vi "Test Find Chessboard Corners.vi"(8 "error in (no error)":errorcluster, 11 "Test Case In":refnum<class "CameraCalibration.lvclass">) -> (0 "error out":errorcluster, 3 "Test Case Out":refnum<class "CameraCalibration.lvclass">)   [LabVIEW 2020, in "g_ar_toolkit.test.lvlib" / "CameraCalibration.lvclass"]
uses:
  CameraCalibration.lvclass
  C:/Program Files (x86)/National Instruments/LabVIEW 2020/vi.lib/Astemes/LUnit/Test Case.lvclass
  g_ar_toolkit.common/Image Point (Float).ctl
  g_ar_toolkit.common/Image Size (Integer).ctl
  g_ar_toolkit.feature_detection/Chessboard Corner Info.ctl
  g_ar_toolkit.image/Interpolation Mode.ctl
  <vilib>/Astemes/LUnit/Test Case.lvclass/Test Case.ctl
  g_ar_toolkit.common/Termination Criteria/Termination Criteria.lvclass/Termination Criteria.ctl
  g_ar_toolkit.image/New Image (Greyscale).vi
  g_ar_toolkit.image/Copy Pixmap to Image (Greyscale Flatten Mask).vi
  g_ar_toolkit.image/Resize (Greyscale).vi
  g_ar_toolkit.feature_detection/FindChessboardCornersGreyscale.vi
  g_ar_toolkit.image/Draw Circle (Greyscale).vi
  g_ar_toolkit.image/Draw Image to Picture (Greyscale).vi
  g_ar_toolkit.image/New Image (Greyscale).vi/6598b9e0-8a08-46f5-91fd-ca1b87217137.vi
  g_ar_toolkit.image/Copy Pixmap to Image (Greyscale Flatten Mask).vi/f0818824-bd55-4656-87f2-fcc208e7cf24.vi
  g_ar_toolkit.image/Resize (Greyscale).vi/eaa3f26c-b51e-4a69-9610-cf2aa5919b39.vi
  g_ar_toolkit.feature_detection/FindChessboardCornersGreyscale.vi/ca99938f-1423-42fb-b653-ffd1f73e2bb5.vi
  <vilib>/Astemes/LUnit/Append Fail Result.vi
  <vilib>/Astemes/LUnit/Append Pass Result.vi
  g_ar_toolkit.common/Termination Criteria/Get Values.vi
  g_ar_toolkit.image/Draw Circle (Greyscale).vi/8336a1cf-e433-4bea-8080-376bdb783d4e.vi
  g_ar_toolkit.image/Draw Image to Picture (Greyscale).vi/9ae995ca-ccda-485c-89ac-02736fde3e8e.vi
  g_ar_toolkit.image/FixPixmap.vi
  <vilib>/Astemes/LUnit/Run In UI.vi
  g_ar_toolkit.image/Default8bitColourMap.vi
  <vilib>/Utility/error.llb/Clear Errors.vi
  <vilib>/picture/picture.llb/Draw Rectangle.vi
  <vilib>/picture/pictutil.llb/Picture to Pixmap.vi
  g_ar_toolkit.common/Module Path.vi
  <vilib>/Utility/error.llb/Error Cluster From Error Code.vi
  g_ar_toolkit.common/Termination Criteria/Termination Criteria.lvclass
  CameraCalibration.lvclass/CameraCalibration.ctl
  g_ar_toolkit.image/g_ar_toolkit.image.lvlib
  g_ar_toolkit.feature_detection/g_ar_toolkit.feature_detection.lvlib
  <vilib>/Astemes/LUnit/Test Case.lvclass
  g_ar_toolkit.common/g_ar_toolkit.common.lvlib
panel:
  out "Points":T1[](array[typedef])
  out "Points Refined":T1[](array[typedef])
  out "Picture":picture
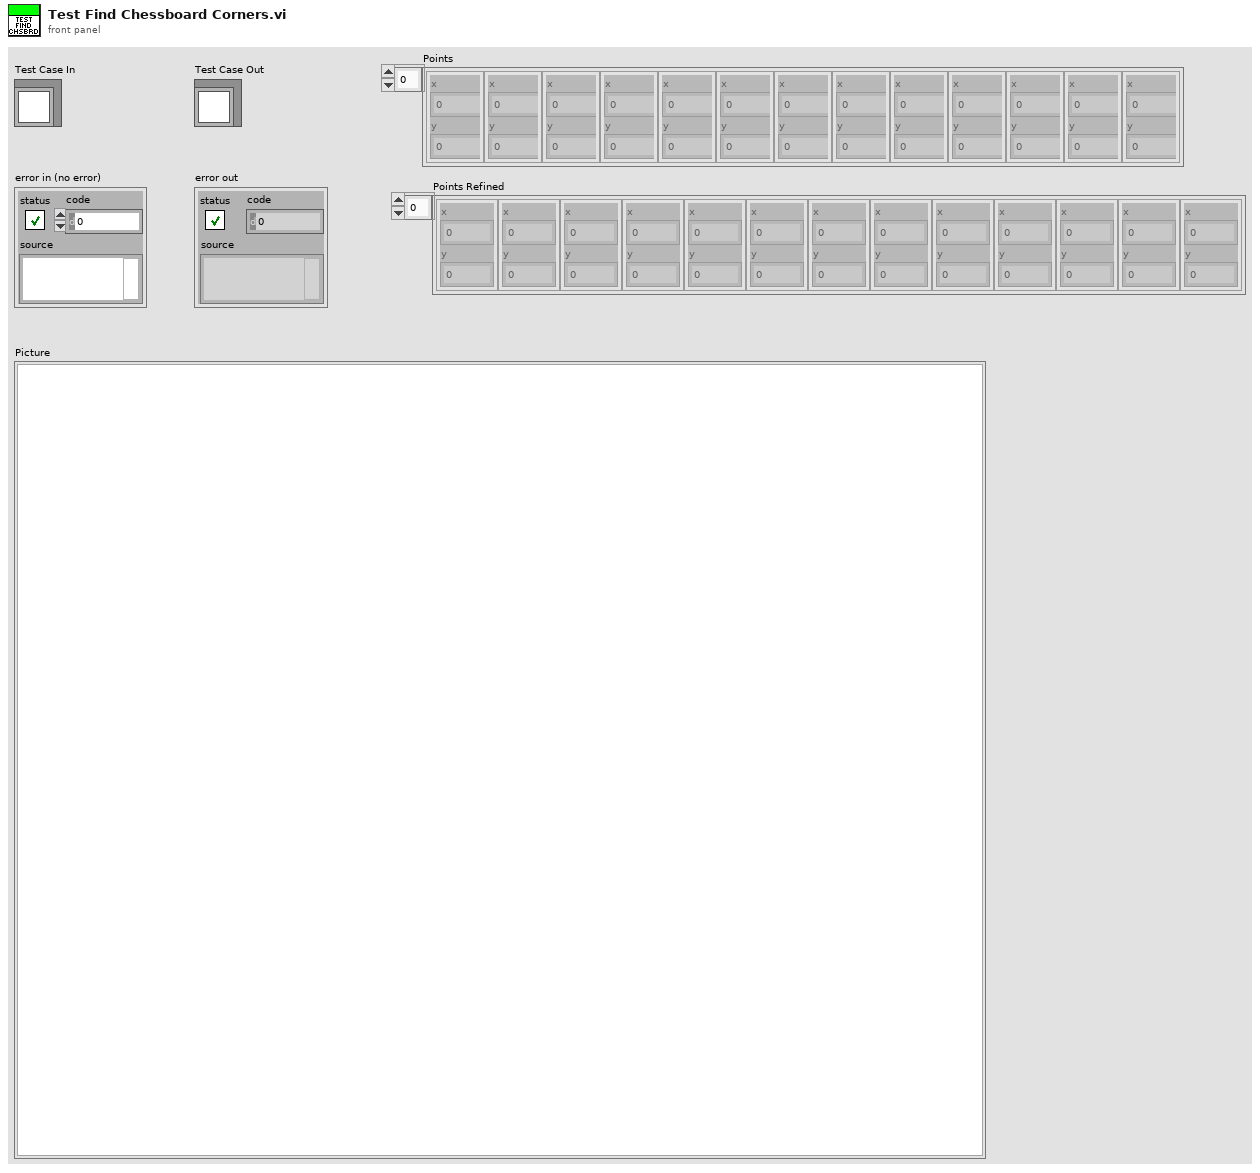
[diagram p1: front panel]
types:
  T1 = typedef "g_ar_toolkit.common.lvlib/Image Point (Float).ctl" = cluster{"x":dbl, "y":dbl}
  T2 = typedef "g_ar_toolkit.image.lvlib/Interpolation Mode.ctl" = enum8{"NEAREST", "LINEAR", "CUBIC", "AREA", "LANCZOS", "LINEAR_EXACT", "NEAREST_EXACT", "MAX"}
  T3 = typedef "g_ar_toolkit.feature_detection.lvlib/Chessboard Corner Info.ctl" = cluster{"Points Per Row":u8, "Points Per Col":u8}
  T4 = typedef "g_ar_toolkit.common.lvlib/Image Size (Integer).ctl" = cluster{"Width":u16, "Height":u16}
  T5 = typedef "imagedata.ctl" = cluster{"image type":i32, "image depth":i32, "image":u8[], "mask":u8[], "colors":u32[], "Rectangle":cluster{"left":i16, "top":i16, "right":i16, "bottom":i16}}
  T6 = typedef "g_ar_toolkit.image.lvlib/Greyscale Image.ctl" = refnum<data-value>
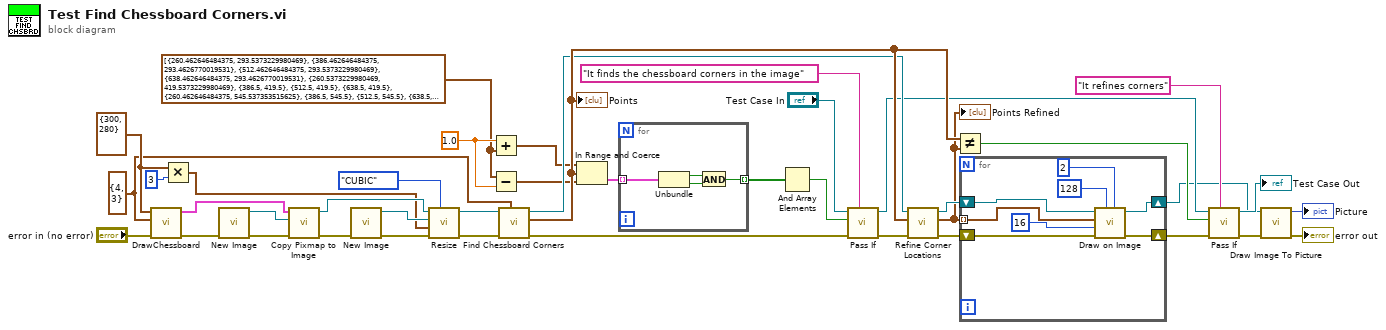
[diagram p0: block diagram]
diagram:
  w2 = T1[] [{"x"=260.462646484375, "y"=293.5373229980469}, {"x"=386.462646484375, "y"=293.4626770019531}, {"x"=512.462646484375, "y"=293.5373229980469}, {"x"=638.462646484375, "y"=293.4626770019531}, {"x"=260.5373229980469, "y"=419.5373229980469}, {"x"=386.5, "y"=419.5}, {"x"=512.5, "y"=419.5}, {"x"=638.5, "y"=419.5}, {"x"=260.462646484375, "y"=545.537353515625}, {"x"=386.5, "y"=545.5}, {"x"=512.5, "y"=545.5}, {"x"=638.5, "y"=545.5}] ("Points")
  w1 = T3 {"Points Per Row"=4, "Points Per Col"=3} ("Chessboard Corners Info")
  w26 = T4 {"Width"=300, "Height"=280} ("Target Size")
  w8 = 1.0
  n1 = call "DrawChessboard.vi"("error in (no error)"="error in (no error)", "Chessboard Corners Info"=w1, "Target Size"=w26) -> ("error out"=w34:errorcluster, "image data"=w35:T5)  [unwired: 7 in]
  n2 = Multiply(x=w26, y=3) -> (x*y=w25:cluster{"Width":i32, "Height":i32})
  n3 = call-poly "New Image.vi"("error in (no error)"=w34) -> ("error out"=w32:errorcluster, "New Greyscale Image"=w36:T6)  [unwired: 9 in]
  n4 = call-poly "Copy Pixmap to Image.vi"("error in (no error)"=w32, "Greyscale Image Destination"=w36, "Pixmap Image Data"=w35) -> ("error out"=w29:errorcluster, "Greyscale Image Destination (duplicate)"=w31:T6)  [unwired: 7 in]
  n5 = call-poly "New Image.vi"("error in (no error)"=w29) -> ("error out"=w28:errorcluster, "New Greyscale Image"=w30:T6)  [unwired: 9 in]
  n6 = call-poly "Resize.vi"("Interpolation Mode (Default: CUBIC)"=Interpolation_Mode."CUBIC" ("OpenCV Interpolation Flag"), "error in (no error)"=w28, "New Image Size"=w25, "Greyscale Destination Image"=w30, "Greyscale Source Image"=w31) -> ("error out"=w27:errorcluster, "Greyscale Destination Image (duplicate)"=w23:T6)  [unwired: 5 in]
  n7 = Add(x=w8, y=w2) -> (x+y=w20:T1[])
  n8 = Subtract(x=w2, y=w8) -> (x-y=w21:T1[])
  n9 = call-poly "Find Chessboard Corners.vi"("Chessboard Corners Info"=w1, "error in (no error)"=w27, "Greyscale Image"=w23) -> ("error out"=w41:errorcluster, "Points"=w40:T1[], "Greyscale Image (Duplicate)"=w37:T6)  [unwired: 6 in]
  "Points" <- w40
  n10 = In Range and Coerce(upper limit=w20, x=w40, lower limit=w21) -> (In Range?=w19:cluster{"x":bool, "y":bool}[])  [unwired: 1 out]
  n11 = for {
    tunnel: w19 -> [w45] mode=indexing
    tunnel: [w42] -> w18 mode=indexing
    n12 = Unbundle(w45) -> ("x"=w44:bool, "y"=w43:bool)
    n13 = And(x=w44, y=w43) -> (x .and. y?=w42:bool)
  }
  n14 = And Array Elements(Boolean array=w18) -> (logical AND=w17:bool)
  n15 = call <vilib>:"Pass If.vi"("Description"="It finds the chessboard corners in the image", "error in (no error)"=w41, "Pass?"=w17, "LUnit Test Case In"="Test Case In") -> ("error out"=w14:errorcluster, "LUnit Test Case Out"=w12:refnum<class "CameraCalibration.lvclass">)  [unwired: 6 in]
  n16 = call "Refine Corner Locations.vi"("error in (no error)"=w14, "Points in"=w40, "Greyscale Image"=w37) -> ("error out"=w6:errorcluster, "Points out"=w3:T1[], "Greyscale Image (Duplicate)"=w7:T6)  [unwired: 6 in]
  "Points Refined" <- w3
  n17 = Not Equal?(x=w40, y=w3) -> (x != y?=w10:bool)
  n18 = for {
    shift-right: [w50] -> w4
    shift-left: w7 -> [w53]
    shift-right: [w51] -> w5
    shift-left: w6 -> [w52]
    tunnel: w3 -> [w49] mode=indexing
    n19 = call-poly "Draw on Image.vi"("Thickness (Default: 1)"=2, "Colour"=u8 128, "error in (no error)"=w52, "Radius"=u16 16, "Centre"=w49, "Greyscale Image"=w53) -> ("error out"=w51:errorcluster, "Greyscale Image (Duplicate)"=w50:T6)  [unwired: 4 in]
  }
  n20 = call <vilib>:"Pass If.vi"("Description"="It refines corners", "error in (no error)"=w5, "Pass?"=w10, "LUnit Test Case In"=w12) -> ("error out"=w13:errorcluster, "LUnit Test Case Out"=→"Test Case Out":refnum<class "CameraCalibration.lvclass">)  [unwired: 6 in]
  n21 = call-poly "Draw Image To Picture.vi"("error in (no error)"=w13, "Greyscale Image Source"=w4) -> ("error out"=→"error out":errorcluster, "Picture"=→"Picture":picture)  [unwired: 8 in]
